vi "SVA 4MV6 P02 CCE RRMA .vi"() -> ()   [LabVIEW 2020]
doc: "Ceballos Conde Emanuel Rodríguez Ramírez Miguel Ángel 4MV6 Sistemas de visión artificial 2022/1\nEste vi da como resultado el color de una region seleccionada de una imagen mediante el uso de un sistema difuso de acuerdo a los lineamientos de la practica P02 de sistemas de vision artificial"
uses:
  SVA 4MV6 P02 CCE RRMA .ctl
  <vilib>/addons/Fuzzy Logic/FL Fuzzy Controller (MISO).vi
  <vilib>/vision/NI_Vision_Development_Module.lvlib
  <vilib>/addons/Fuzzy Logic/NI_Fuzzy_Logic_API.lvlib
panel:
  out "B":u8
  out "G":u8
  out "R":u8
  out "Color promedio":u32(colorbox)
  in  "Sistema difuso":path
  in  "Tamaño (pixeles)":i32=50
  out "Muestra":T1(plugin-control)
  out "Color sistema difuso":u32(colorbox)
  in  "Imagen":path
  in  "stop":bool
  out "Imagen":T1(plugin-control)
  # "Ceballos Conde Emanuel\nRodríguez Ramírez Miguel Ángel\n4MV6\nSistemas de visión artificial\n2022/1"
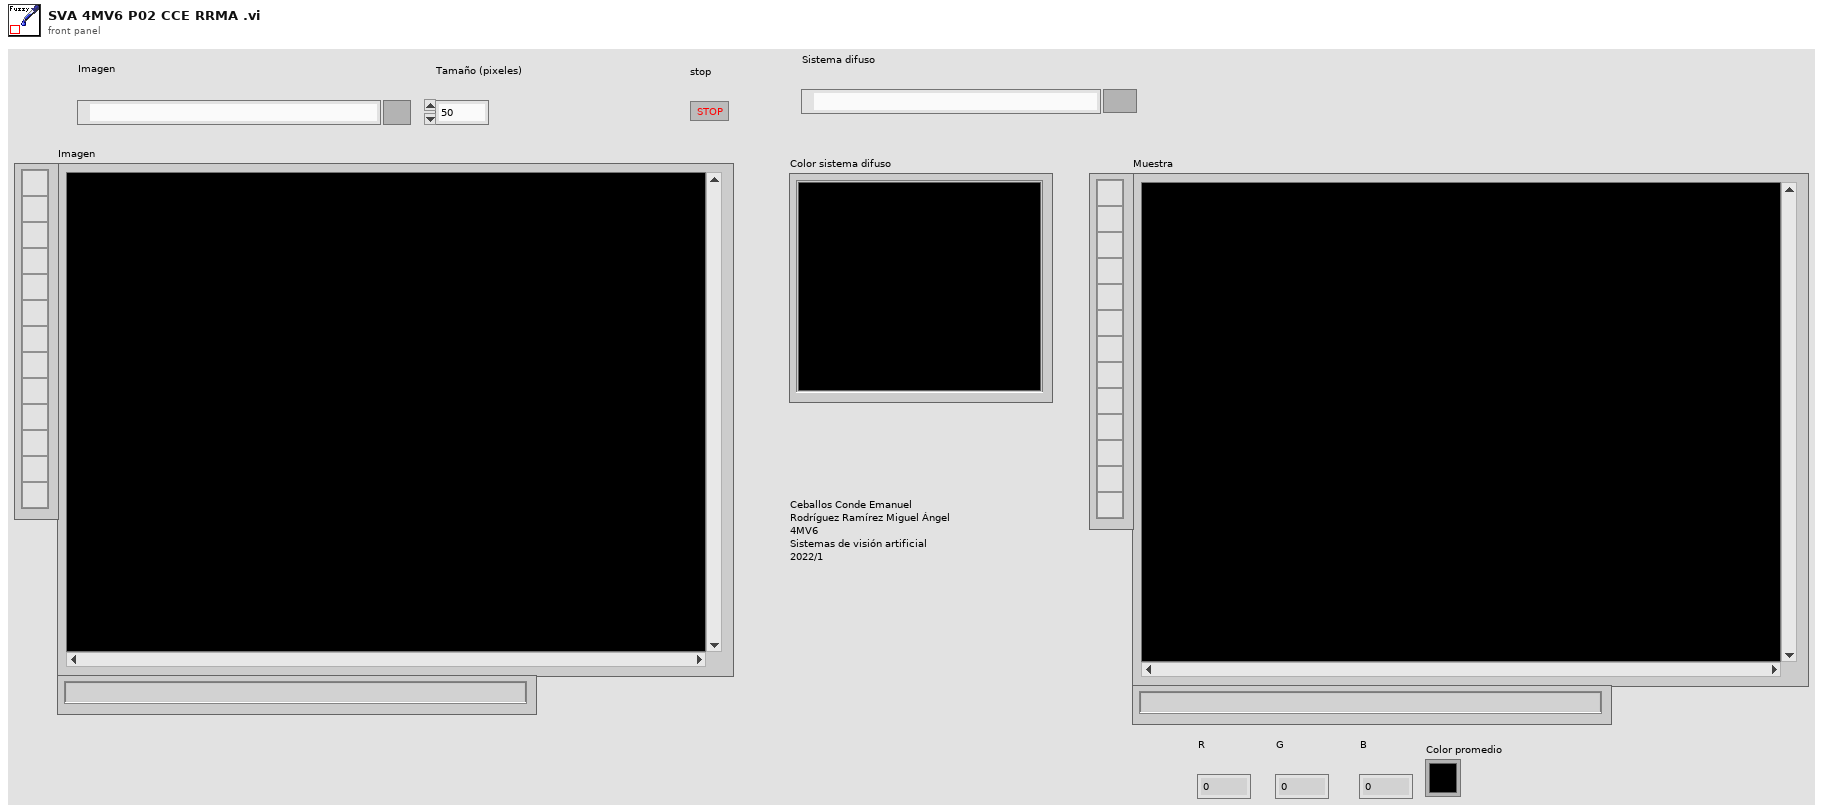
[diagram p1: front panel]
types:
  T1 = typedef "IMAQ Image.ctl" = refnum<image>
  T2 = typedef "Image Type" = u32
  T3 = typedef "SVA 4MV6 P02 CCE RRMA .ctl" = enum16{"Espera", "muestra", "color"}
  T4 = typedef "NI_Fuzzy_Logic_API.lvlib/FL System.ctl" = cluster{"input variables":T5[], "output variables":T5[], "rules":T8[], "defuzzification method":T14, "description":string, "user MF interpolating polynomials":T15[]}
  T5 = typedef "NI_Fuzzy_Logic_API.lvlib/FL Variable.ctl" = cluster{"name":string, "range":dbl[], "MFs":T6[]}
  T6 = typedef "NI_Fuzzy_Logic_API.lvlib/FL Membership Function.ctl" = cluster{"name":string, "shape":T7, "points":dbl[], "color":u32, "user-defined shape index":i32}
  T7 = typedef "NI_Fuzzy_Logic_API.lvlib/FL Membership Function Shape.ctl" = u16
  T8 = typedef "NI_Fuzzy_Logic_API.lvlib/FL Rule.ctl" = cluster{"antecedents":T9[], "antecedent connective":T11, "consequents":T12[], "consequent implication":T13, "degree of support":dbl}
  T9 = typedef "NI_Fuzzy_Logic_API.lvlib/FL Antecedent.ctl" = cluster{"Var Index":i32, "MF Index":i32, "Cond":T10}
  T10 = typedef "NI_Fuzzy_Logic_API.lvlib/FL Modifier.ctl" = u16
  T11 = typedef "NI_Fuzzy_Logic_API.lvlib/FL Antecedent Connective.ctl" = u16
  T12 = typedef "NI_Fuzzy_Logic_API.lvlib/FL Consequent.ctl" = cluster{"Var Index":i32, "MF Index":i32, "Cond":T10}
  T13 = typedef "NI_Fuzzy_Logic_API.lvlib/FL Consequent Implication.ctl" = u16
  T14 = typedef "NI_Fuzzy_Logic_API.lvlib/FL Defuzzification.ctl" = u16
  T15 = typedef "NI_Fuzzy_Logic_API.lvlib/FL Interpolating polynomials.ctl" = cluster{"X":dbl[], "Y":dbl[], "Y(x) coeff":dbl[][], "X(y) coeff":dbl[][], "Area(y) coeff":dbl[][], "coa_x(y) coeff":dbl[][]}
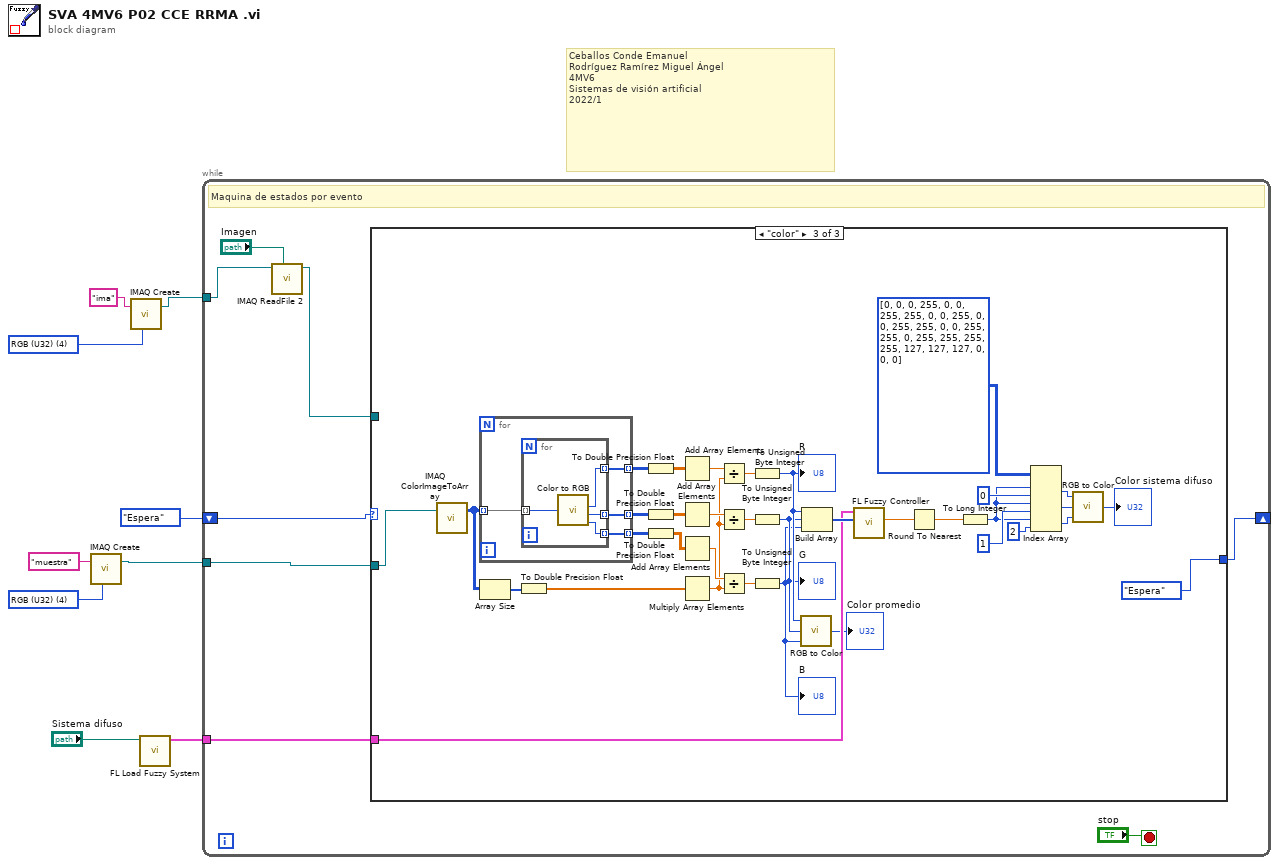
[diagram p0: block diagram]
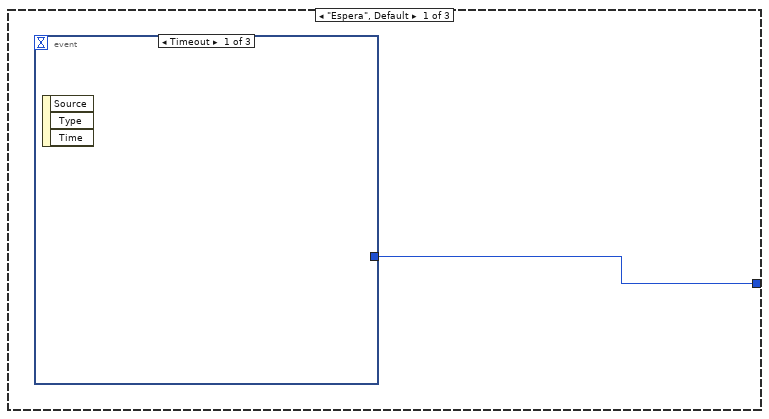
[diagram p2: hidden frame]
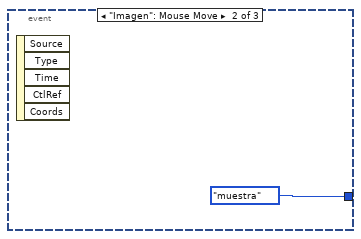
[diagram p3: hidden frame]
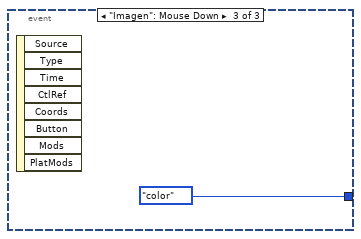
[diagram p4: hidden frame]
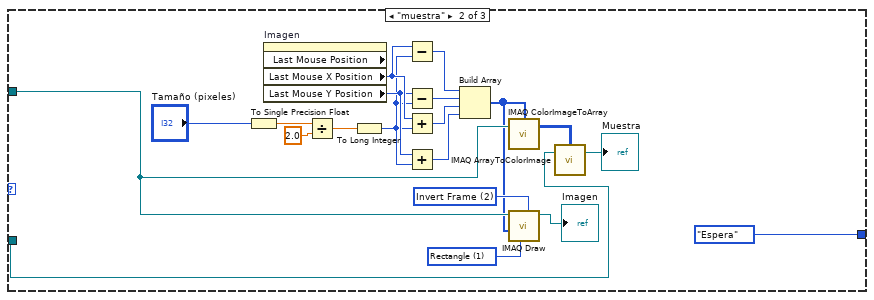
[diagram p5: hidden frame]
diagram:
  w6 = T2 4 items=["Grayscale (U8)", "Grayscale (I16)", "Grayscale (SGL)", "Complex (CSG)", "RGB (U32)", "HSL (U32)", "RGB (U64)", "Grayscale (U16)"] ("Image Type")
  w7 = T2 4 items=["Grayscale (U8)", "Grayscale (I16)", "Grayscale (SGL)", "Complex (CSG)", "RGB (U32)", "HSL (U32)", "RGB (U64)", "Grayscale (U16)"] ("Image Type")
  # "Ceballos Conde Emanuel\nRodríguez Ramírez Miguel Ángel\n4MV6\nSistemas de visión artificial\n2022/1"
  n1 = call "IMAQ Create"("Image Name"="muestra", "Image Type"=w6) -> ("New Image"=w4:T1)  [unwired: 3 in, 1 out]
  n2 = call "IMAQ Create"("Image Name"="ima", "Image Type"=w7) -> ("New Image"=w3:T1)  [unwired: 3 in, 1 out]
  n3 = call <vilib>:"FL Load Fuzzy System.vi"("file path"="Sistema difuso") -> ("fuzzy system out"=w1:T4)  [unwired: 9 in, 1 out]
  n4 = while {
    shift-right: [w10] -> _
    shift-left: SVA_4MV6_P02_CCE_RRMA_."Espera" -> [w17]
    tunnel: w4 -> [w15]
    tunnel: w3 -> [w14]
    tunnel: w1 -> [w11]
    stop <- "stop" stop-if-true
    # "Maquina de estados por evento"
    n5 = call "IMAQ ReadFile 2"("File Path"="Imagen", "Image"=w14) -> ("Image Out"=w13:T1)  [unwired: 5 in, 4 out]
    n6 = case shown="\"color\"" w17 {
      tunnel: [w18 SVA_4MV6_P02_CCE_RRMA_."Espera" SVA_4MV6_P02_CCE_RRMA_."Espera"] -> w10
      tunnel: w13 -> [_ w30 _]
      tunnel: w15 -> [_ w28 w75]
      tunnel: w11 -> [_ _ w49]
      frame "Espera", Default {
        n7 = event shown="[0] Timeout" {
          selector: _ -> [_ _ _]
          dyn-events: _ -> [_ _ _]
          timeout: _ -> [_ _ _]
          tunnel: [_ SVA_4MV6_P02_CCE_RRMA_."muestra" SVA_4MV6_P02_CCE_RRMA_."color"] -> w18
          event Timeout {
            n8 = event-data() -> ()  [unwired: 1 in, 3 out]
          }
          event "Imagen": Mouse Move {
            n9 = event-data() -> ()  [unwired: 1 in, 5 out]
          }
          event "Imagen": Mouse Down {
            n10 = event-data() -> ()  [unwired: 1 in, 8 out]
          }
        }
      }
      frame "muestra" {
        w38 = u16 2 items=["Frame", "Paint", "Invert Frame", "Invert Paint"] ("Draw Mode")
        w39 = u16 1 items=["Line", "Rectangle", "Oval"] ("Shape to draw")
        n11 = To Single Precision Float(number="Tamaño (pixeles)") -> (single precision float=w23:sgl)
        n12 = property on="Imagen" class="ImageControl" props=["Last Mouse Position", "Last Mouse X Position", "Last Mouse Y Position"]() -> ("Last Mouse X Position"=w37:i32, "Last Mouse Y Position"=w36:i32)  [unwired: 2 in, 3 out]
        n13 = Divide(x=w23, y=sgl 2.0) -> (x/y=w26:sgl)
        n14 = To Long Integer(number=w26) -> (32bit integer=w22:i32)
        n15 = Subtract(x=w37, y=w22) -> (x-y=w35:i32)
        n16 = Subtract(x=w36, y=w22) -> (x-y=w34:i32)
        n17 = Add(x=w37, y=w22) -> (x+y=w33:i32)
        n18 = Add(x=w36, y=w22) -> (x+y=w32:i32)
        n19 = Build Array(w35, w34, w33, w32) -> (w29:i32[])
        n20 = call "IMAQ ColorImageToArray"("Optional Rectangle"=w29, "Image"=w30) -> ("Image Pixels (U32)"=w21:u32[][])  [unwired: 2 in, 2 out]
        n21 = call "IMAQ Draw"("Draw Mode"=w38, "Shape to draw"=w39, "Coordinates"=w29, "Image Src"=w30) -> ("Image Dst Out"=→"Imagen":T1)  [unwired: 6 in, 1 out]
        n22 = call "IMAQ ArrayToColorImage"("Image Pixels (U32)"=w21, "Image"=w28) -> ("Image Out"=→"Muestra":T1)  [unwired: 3 in, 1 out]
      }
      frame "color" {
        n23 = call "IMAQ ColorImageToArray"("Image"=w75) -> ("Image Pixels (U32)"=w71:u32[][])  [unwired: 3 in, 2 out]
        n24 = for {
          tunnel: w71 -> [w79] mode=indexing
          tunnel: [w76] -> w74 mode=indexing
          tunnel: [w78] -> w60 mode=indexing
          tunnel: [w77] -> w59 mode=indexing
          n25 = for {
            tunnel: w79 -> [w83] mode=indexing
            tunnel: [w82] -> w76 mode=indexing
            tunnel: [w81] -> w78 mode=indexing
            tunnel: [w80] -> w77 mode=indexing
            n26 = call <vilib>:"Color to RGB.vi"("Color"=w83) -> ("R"=w82:u8, "G"=w81:u8, "B"=w80:u8)  [unwired: 1 out]
          }
        }
        n27 = Array Size(array=w71) -> (size(s)=w70:i32[])
        n28 = To Double Precision Float(number=w70) -> (double precision float=w69:dbl[])
        n29 = To Double Precision Float(number=w74) -> (double precision float=w73:dbl[][])
        n30 = To Double Precision Float(number=w60) -> (double precision float=w66:dbl[][])
        n31 = To Double Precision Float(number=w59) -> (double precision float=w65:dbl[][])
        n32 = Add Array Elements(numeric array=w73) -> (sum=w72:dbl)
        n33 = Add Array Elements(numeric array=w66) -> (sum=w67:dbl)
        n34 = Add Array Elements(numeric array=w65) -> (sum=w64:dbl)
        n35 = Multiply Array Elements(1:w69) -> (0:w63:dbl)
        n36 = Divide(x=w72, y=w63) -> (x/y=w68:dbl)
        n37 = Divide(x=w67, y=w63) -> (x/y=w62:dbl)
        n38 = Divide(x=w64, y=w63) -> (x/y=w61:dbl)
        n39 = To Unsigned Byte Integer(number=w68) -> (unsigned 8bit integer=w46:u8)
        "R" <- w46
        n40 = To Unsigned Byte Integer(number=w62) -> (unsigned 8bit integer=w45:u8)
        "G" <- w45
        n41 = To Unsigned Byte Integer(number=w61) -> (unsigned 8bit integer=w44:u8)
        "B" <- w44
        n42 = call <vilib>:"RGB to Color.vi"("B"=w44, "G"=w45, "R"=w46) -> ("Color"=→"Color promedio":u32)
        n43 = Build Array(w46, w45, w44) -> (w58:u8[])
        n44 = call-poly <vilib>:"FL Fuzzy Controller.vi"("input values"=w58, "fuzzy system in"=w49) -> ("output value"=w57:dbl)  [unwired: 5 in, 4 out]
        n45 = Round To Nearest(number=w57) -> (nearest integer value=w42:dbl)
        n46 = To Long Integer(number=w42) -> (32bit integer=w41:i32)
        n47 = Index Array(array=u8[][] [[0, 0, 0], [255, 0, 0], [255, 255, 0], [0, 255, 0], [0, 255, 255], [0, 0, 255], [255, 0, 255], [255, 255, 255], [127, 127, 127], [0, 0, 0]], index (row) #1=w41, index (col) #1=0 ("disabled index (col)"), index (row) #2=w41, index (col) #2=1 ("index (col)"), index (row) #3=w41, index (col) #3=2 ("index (col)")) -> (element #1=w52:u8, element #2=w51:u8, element #3=w50:u8)
        n48 = call <vilib>:"RGB to Color.vi"("B"=w50, "G"=w51, "R"=w52) -> ("Color"=→"Color sistema difuso":u32)
      }
    }
  }
